vi "TableCollum(SubVI).vi"(10 "ScaleOrdinate 2":T1(ring)=enum."Проценты" caption="Ось ординат", 11 "UNDT_NTick":i32) -> (3 "array":string[][](array[string]))   [LabVIEW 2017]
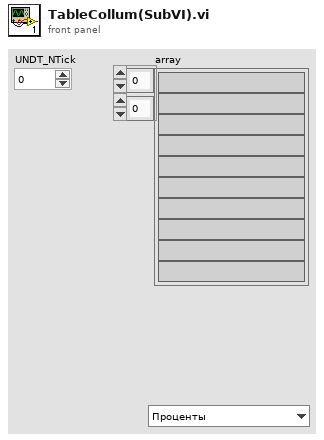
[diagram p1: front panel]
types:
  T1 = enum16{"Отсчеты АЦП (±32767)", "Проценты", "Вольты", "дБмкВ (отн. 1 мкВ)", "Отсчеты АЦП (±1)"}
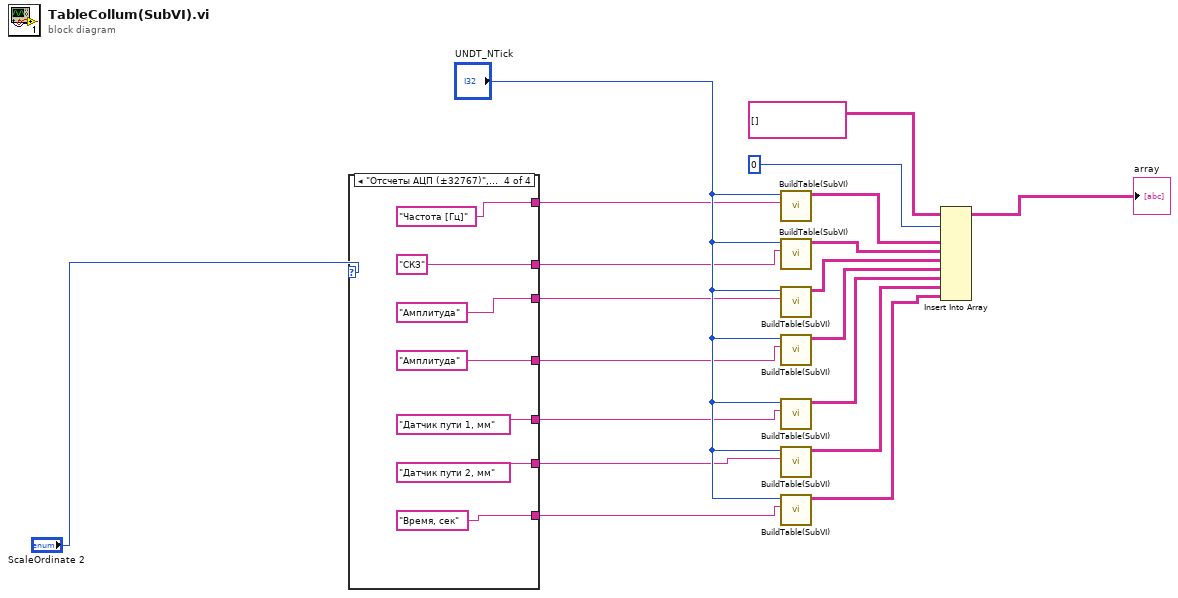
[diagram p0: block diagram]
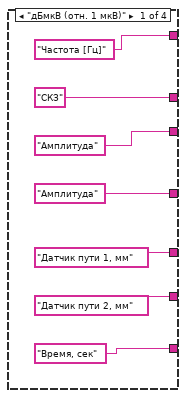
[diagram p2: hidden frame]
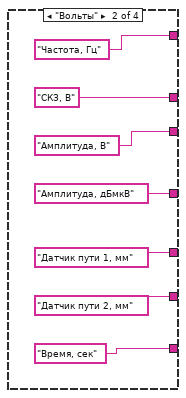
[diagram p3: hidden frame]
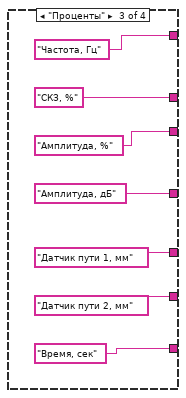
[diagram p4: hidden frame]
diagram:
  n1 = case shown="\"Отсчеты АЦП (±32767)\", Default" "ScaleOrdinate 2" {
    tunnel: ["Амплитуда" "Амплитуда, дБмкВ" "Амплитуда, дБ" "Амплитуда"] -> w8
    tunnel: ["Время, сек" "Время, сек" "Время, сек" "Время, сек"] -> w7
    tunnel: ["Датчик пути 2, мм" "Датчик пути 2, мм" "Датчик пути 2, мм" "Датчик пути 2, мм"] -> w6
    tunnel: ["Датчик пути 1, мм" "Датчик пути 1, мм" "Датчик пути 1, мм" "Датчик пути 1, мм"] -> w5
    tunnel: ["Частота [Гц]" "Частота, Гц" "Частота, Гц" "Частота [Гц]"] -> w4
    tunnel: ["Амплитуда" "Амплитуда, В" "Амплитуда, %" "Амплитуда"] -> w3
    tunnel: ["СКЗ" "СКЗ, В" "СКЗ, %" "СКЗ"] -> w2
    frame "дБмкВ (отн. 1 мкВ)" {
    }
    frame "Вольты" {
    }
    frame "Проценты" {
    }
    frame "Отсчеты АЦП (±32767)", Default {
    }
  }
  n2 = call "BuildTable(SubVI).vi"("String"=w4, "UNDT_NTick"="UNDT_NTick") -> ("Array"=w17:string[][])  [unwired: 9 in]
  n3 = call "BuildTable(SubVI).vi"("String"=w2, "UNDT_NTick"="UNDT_NTick") -> ("Array"=w14:string[][])  [unwired: 9 in]
  n4 = call "BuildTable(SubVI).vi"("String"=w3, "UNDT_NTick"="UNDT_NTick") -> ("Array"=w19:string[][])  [unwired: 9 in]
  n5 = call "BuildTable(SubVI).vi"("String"=w8, "UNDT_NTick"="UNDT_NTick") -> ("Array"=w9:string[][])  [unwired: 9 in]
  n6 = call "BuildTable(SubVI).vi"("String"=w5, "UNDT_NTick"="UNDT_NTick") -> ("Array"=w10:string[][])  [unwired: 9 in]
  n7 = call "BuildTable(SubVI).vi"("String"=w6, "UNDT_NTick"="UNDT_NTick") -> ("Array"=w11:string[][])  [unwired: 9 in]
  n8 = call "BuildTable(SubVI).vi"("String"=w7, "UNDT_NTick"="UNDT_NTick") -> ("Array"=w12:string[][])  [unwired: 9 in]
  n9 = Insert Into Array(array=string[][] [], index (row)=0, new element #1=w17, new element #2=w14, new element #3=w19, new element #4=w9, new element #5=w10, new element #6=w11, new element #7=w12) -> (→"array":string[][])  [unwired: 1 in]
